vi "SIM update backward differences.vi"(10 "New y":dbl[](array[numeric]), 11 "Backward differences":dbl[][](array[numeric])) -> (2 "New y out":dbl[](array[numeric]), 3 "New Backward differences":dbl[][](array[numeric]))   [LabVIEW 2017]
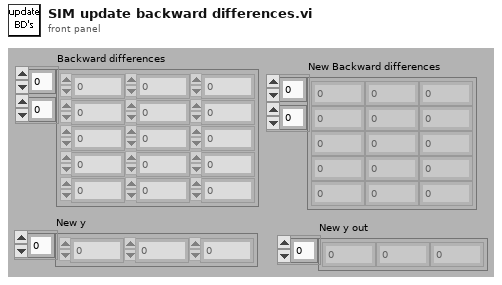
[diagram p1: front panel]
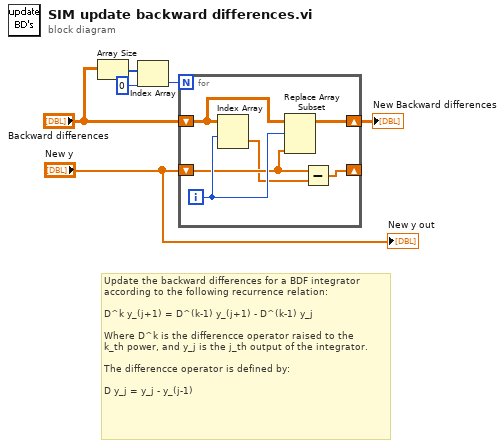
[diagram p0: block diagram]
diagram:
  # "Update the backward differences for a BDF integrator\naccording to the following recurrence relation:\n\nD^k y_(j+1) = D^(k-1) y_(j+1) - D^(k-1) y_j\n\nWhere D^k is the differencce operator raised to the\nk_th power, and y_j is the j_th output of the integrator.\n\nThe differencce operator is defined by:\n\nD y_j = y_j - y_(j-1)"
  n1 = Array Size(array="Backward differences") -> (size(s)=w4:i32[])
  n2 = Index Array(array=w4, index=0) -> (element=w2:i32)
  n3 = for {
    N: w2 -> [_]
    shift-right: [w10] -> w6
    shift-left: "Backward differences" -> [w12]
    shift-right: [w8] -> _
    shift-left: "New y" -> [w9]
    i -> [w11]
    n4 = Index Array(array=w12, index (row)=w11) -> (element=w7:dbl[])  [unwired: 1 in]
    n5 = Replace Array Subset(array=w12, new element=w9, index (row)=w11) -> (w10:dbl[][])  [unwired: 1 in]
    n6 = Subtract(x=w9, y=w7) -> (x-y=w8:dbl[])
  }
  "New Backward differences" <- w6
  "New y out" <- "New y"
